vi "Set Oscillator Sweep.vi"(8 "error in (no error)":errorcluster, 10 "Frequency and Amplitude Control":T1, 11 "VISA resource name":refnum<visa-resource-name>) -> (0 "error out":errorcluster, 3 "VISA resource name out":refnum<visa-resource-name>)   [LabVIEW 2016, in "SR7270 Drivers.lvlib"]
uses:
  SR7270 Drivers.lvlib
  Typedefs/SWEEP--enum.ctl
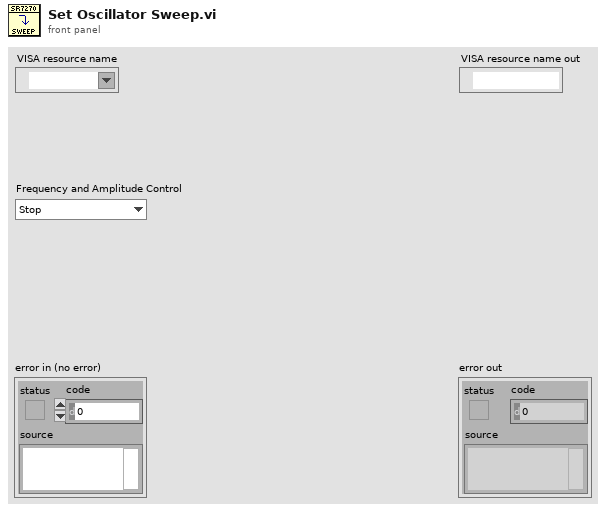
[diagram p1: front panel]
types:
  T1 = typedef "SR7270 Drivers.lvlib/SWEEP--enum.ctl" = enum16{"Stop", "Start/continue f sweep", "Start/continue A sweep", "Start/continue f&A sweep", "n/a (4)", "Pause f sweep", "Pause A sweep", "Pause f&A sweep", "n/a (8)", "Link f sweep to CB", "Link A sweep to CB", "Link f&A sweep to CB"}
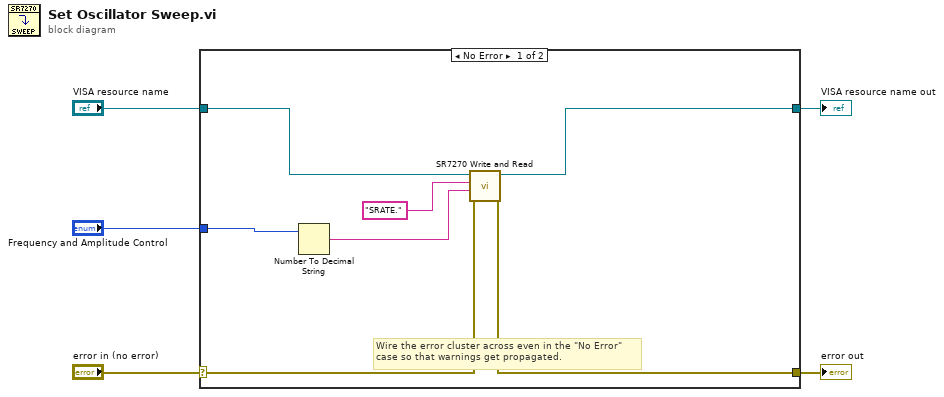
[diagram p0: block diagram]
diagram:
  n1 = case shown="No Error" "error in (no error)" {
    selector: "error in (no error)" -> [w12 w14]
    tunnel: [w11 w14] -> w4
    tunnel: [w6 w13] -> w2
    tunnel: "VISA resource name" -> [w7 w13]
    tunnel: "Frequency and Amplitude Control" -> [w10 _]
    frame No Error {
      # "Wire the error cluster across even in the \"No Error\"\ncase so that warnings get propagated."
      n2 = Number To Decimal String(number=w10) -> (decimal integer string=w8:string)  [unwired: 1 in]
      n3 = call "SR7270 Write and Read.vi"("error in (no error)"=w12, "Parameter(s)"=w8, "Command Name"="SRATE.", "VISA resource name"=w7) -> ("error out"=w11:errorcluster, "VISA resource name out"=w6:refnum<visa-resource-name>)  [unwired: 4 in, 2 out]
    }
    frame Error {
    }
  }
  "error out" <- w4
  "VISA resource name out" <- w2
